vi "Test Parse Date String.vi"(8 "error in (no error)":errorcluster, 11 "Test Case In":refnum<class "Barcode Type A Test.lvclass">) -> (0 "error out":errorcluster, 3 "Test Case Out":refnum<class "Barcode Type A Test.lvclass">)   [LabVIEW 2020, in "Barcode Reader Second Iteration.lvlib" / "Barcode Type A Test.lvclass"]
uses:
  Barcode Type A Test.lvclass
  C:/Program Files (x86)/National Instruments/LabVIEW 2020/vi.lib/Astemes/LUnit/Test Case.lvclass
  <vilib>/Astemes/LUnit/Test Case.lvclass/Test Case.ctl
  01074fa8-ee8a-411d-bc8b-fc92c4f90959.vi
  <vilib>/Astemes/LUnit/Palette/Pass.vi
  <vilib>/Astemes/LUnit/Palette/Fail.vi
  <vilib>/Astemes/LUnit/Compare Variants.vi
  <vilib>/Astemes/LUnit/Describe Comparison.vi
  <vilib>/Astemes/LUnit/Set Assertion Type.vi
  <vilib>/Astemes/LUnit/Add test result.vi
  <vilib>/Astemes/LUnit/Variant to string.vi
  <vilib>/Astemes/LUnit/LUnit Record Assertion Result.vi
  <vilib>/Astemes/LUnit/LUnit Aggregate Assertion Results.vi
  <vilib>/Astemes/LUnit/Method Result/LUnit Merge Status.vi
  <vilib>/Astemes/LUnit/LUnit Concatenate result strings.vi
  <vilib>/Utility/Data Type/Get Type Information.vi
  <vilib>/Utility/LVClass/Get LV Class Name.vi
  Barcode Reader/Barcode.lvclass
  Barcode Type A Test.lvclass/Barcode Type A Test.ctl
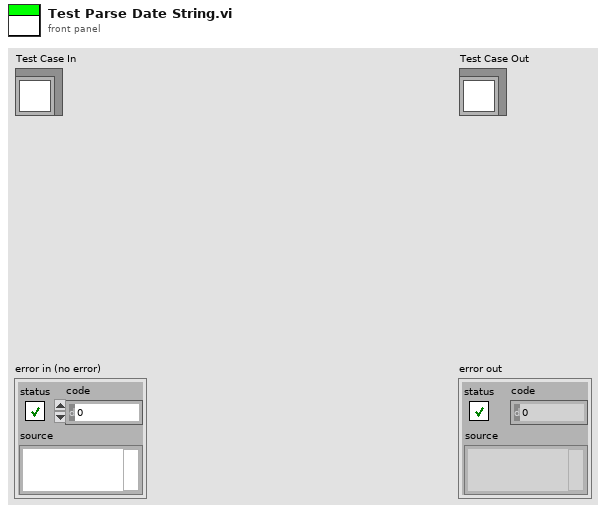
[diagram p1: front panel]
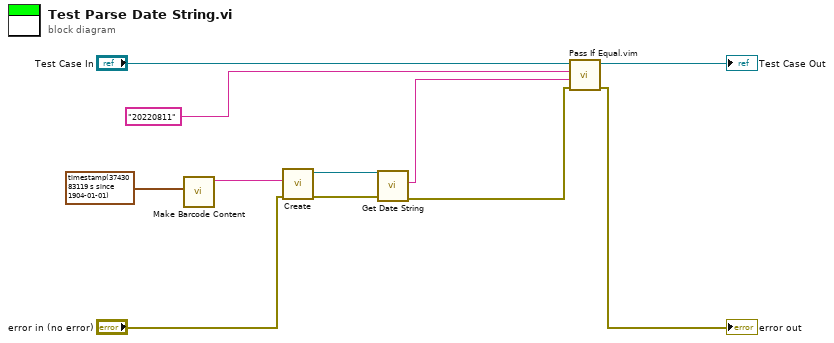
[diagram p0: block diagram]
diagram:
  n1 = call "Make Barcode Content.vi"("Date"=timestamp(3743083119.3780074 s since 1904-01-01)) -> ("Barcode Content"=w8:string)  [unwired: 10 in]
  n2 = call "Create.vi"("error in (no error)"="error in (no error)", "Barcode Content"=w8) -> ("error out"=w5:errorcluster, "Barcode Reader Out"=w7:refnum<class "Barcode.lvclass">)  [unwired: 8 in]
  n3 = call-dynamic "Get Date String.vi"("error in (no error)"=w5, "Barcode Reader in"=w7) -> ("error out"=w3:errorcluster, "Date String"=w6:string)  [unwired: 7 in, 1 out]
  n4 = call "Pass If Equal.vim"("error in (no error)"=w3, "Actual"=w6, "Expected"="20220811", "LUnit Test Case In"="Test Case In") -> ("error out"=→"error out":errorcluster, "LUnit Test Case Out"=→"Test Case Out":refnum<class "Barcode Type A Test.lvclass">)  [unwired: 6 in]
